vi "MCSA Spectra (1 Motor with IC).vi"(0 "waveforms":waveform(dbl)[](array[waveform]), 2 "reset? (F)":bool, 7 "spectrum settings":T5={"number of lines"=15000, "% overlap"=0.0, "maximum frequency [Hz]"=250.0}, 9 "initial conditions":T1 {"zoom FFT settings"."FFT settings"."window" items=["Rectangle"=0, "Hanning"=1, "Hamming"=2, "Blackman-Harris"=3, "Exact Blackman"=4, "Blackman"=5, "Flat Top"=6, "4 Term B-Harris "=7, "7 Term B-Harris"=8, "Low Sidelobe"=9, "Blackman Nuttall"=11, "Triangle"=30, "Bartlett-Hanning"=31, "Bohman"=32, "Parzen"=33, "Welch"=34, "Kaiser"=60, "Dolph-Chebyshev"=61, "Gaussian"=62]}, 11 "error in (no error)":errorcluster, 12 "demodulation settings":cluster{"enable? (F)":bool, "algorithm":T2}={"enable? (F)"=FALSE, "algorithm"=enum."3-phase signals"}) -> (3 "new spectrum available?":bool, 4 "spectrum information":T4, 10 "final conditions":T1 {"zoom FFT settings"."FFT settings"."window" items=["Rectangle"=0, "Hanning"=1, "Hamming"=2, "Blackman-Harris"=3, "Exact Blackman"=4, "Blackman"=5, "Flat Top"=6, "4 Term B-Harris "=7, "7 Term B-Harris"=8, "Low Sidelobe"=9, "Blackman Nuttall"=11, "Triangle"=30, "Bartlett-Hanning"=31, "Bohman"=32, "Parzen"=33, "Welch"=34, "Kaiser"=60, "Dolph-Chebyshev"=61, "Gaussian"=62]}, 15 "error out":errorcluster)   [LabVIEW 2014, in "NI_EP_Motor Monitoring.lvlib"]
doc: "Calculates the zoom fast Fourier Transform (FFT) spectra of the motor. You must manually select the polymorphic instance you want to use."
uses:
  <vilib>/addons/Electrical Power/Motor Monitoring/NI_EP_Motor Monitoring.lvlib
  <vilib>/addons/Electrical Power/Motor Monitoring/subVIs/ep_Spectra Settings.ctl
  <vilib>/addons/Electrical Power/Motor Monitoring/subVIs/ep_Demodulation Algorithm.ctl
  <vilib>/addons/Electrical Power/Motor Monitoring/subVIs/ep_Initial Conditions for MCSA Spectra.ctl
  <vilib>/addons/Electrical Power/Motor Monitoring/subVIs/ep_Zoom FFT Settings.ctl
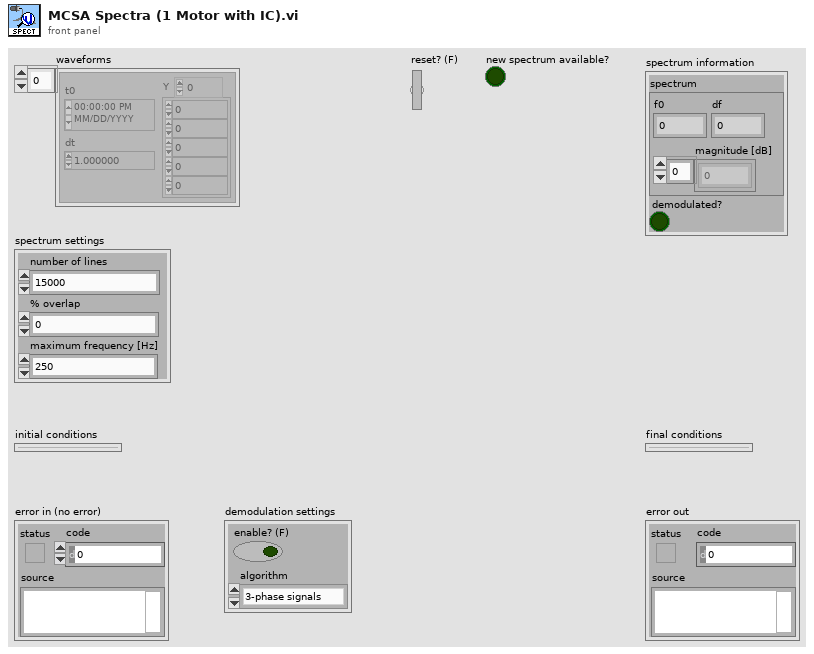
[diagram p1: front panel]
types:
  T1 = typedef "NI_EP_Motor Monitoring.lvlib/ep_Initial Conditions for MCSA Spectra.ctl" = cluster{"hilbert state":cluster{"delay conditions":dbl[], "filter conditions":dbl[]}, "zoom FFT state":cluster{"phase state":dbl, "zoom FFT state":cluster{"zoom settings state":cluster{"zoom":i32, "stop band attenuation":enum16{"84 dB", "96 dB", "120 dB"}, "alias protect in final transition":bool, "oversampling ratio":dbl}, "SML Decimation Filter (complex input) state":cluster{"decimation settings state":cluster{"M":i32, "stop band attenuation":enum16{"84 dB", "96 dB", "120 dB"}, "alias protect in transition band":bool, "oversampling ratio":dbl}, "counter for garbage samples state":i32, "sml_Parameter Setting for Zoom Factor state":cluster{"filter length * interpolation state":i32, "interpolation state":i32, "comb filter order state":i32, "CFIR par state":cluster{"h":dbl[], "M":i32, "N":i32}, "LFIR par state":cluster{"h":dbl[], "M":i32, "N":i32}, "CIC Stages state":i32}, "aal_CIC (complex input) state":cluster{"aal_cascaded moving average (complex input) state":cluster{"states":cdb[], "circular buffers state":cdb[][], "circular buffer counter state":i32}, "aal_moving average with decimation by order (complex input) state":cluster{"residue result state":cdb, "processed data counter state":i32}}, "sml_Cascaded Decimation Filter (complex input) CFIR state":cluster{"unprocessed data state":cdb[], "final conditions state":cdb[][], "sml_M-1 Decimator with IC (complex input) state":cluster{"coefficients in reverse order state":dbl[], "max index for coefficients state":i32}}, "sml_Cascaded Decimation Filter (complex input) LFIR state":cluster{"unprocessed data state":cdb[], "final conditions state":cdb[][], "sml_M-1 Decimator with IC (complex input) state":cluster{"coefficients in reverse order state":dbl[], "max index for coefficients state":i32}}}, "ma_SML Data Packing (complex input) state":cluster{"array getting packed state":cdb[], "last array processed state":cdb[], "index state":i32, "packing parameters state":cluster{i32, "size":i32}}}, "FFT{X} [Vrms]":cdb[]}, "IIR filter state":cluster{"filter state":dbl[]}, "demodulation settings":cluster{"enable? (F)":bool, "algorithm":T2}, "highpass IIR Filter":cluster{"filter structure":enum32{"IIR 2nd Order", "IIR 4th Order"}, "Reverse Coefficients":dbl[], "Forward Coefficients":dbl[]}, "Hilbert FIR filter":cluster{"coefficients":dbl[], "delay":i32}, "zoom FFT settings":T3}
  T2 = typedef "NI_EP_Motor Monitoring.lvlib/ep_Demodulation Algorithm.ctl" = enum16{"1-phase signal", "3-phase signals"}
  T3 = typedef "NI_EP_Motor Monitoring.lvlib/ep_Zoom FFT Settings.ctl" = cluster{"FFT settings":cluster{"window":u16, "Window Size":i32, "FFT Size":i32, "%overlap":dbl}, "zoom settings":cluster{"zoom":i32, "stop band attenuation":enum16{"84 dB", "96 dB", "120 dB"}, "alias protect in final transition":bool, "oversampling ratio":dbl}, "other settings":cluster{"fmod":dbl, "f0":dbl, "df":dbl, "oidx":i32, "olen":i32}, "iterations":i32, "max block size":i32, "fs":dbl}
  T4 = cluster{"spectrum":cluster{"f0":dbl, "df":dbl, "magnitude [dB]":dbl[]}, "demodulated?":bool}
  T5 = typedef "NI_EP_Motor Monitoring.lvlib/ep_Spectra Settings.ctl" = cluster{"number of lines":i32, "% overlap":dbl, "maximum frequency [Hz]":dbl}
  T6 = cluster{"spectra":cluster{"f0":dbl, "df":dbl, "magnitude [dB]":dbl[]}, "demodulated?":bool}
  T7 = cluster{"demodulation settings":cluster{"enable? (F)":bool, "algorithm":T2}, "dt":dbl, "block size":i32}
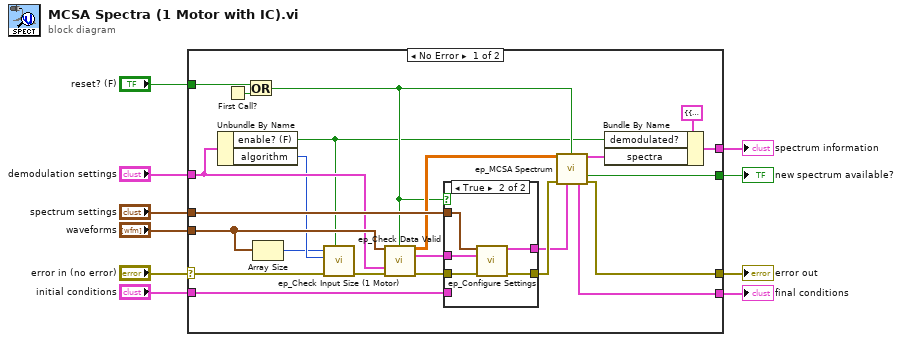
[diagram p0: block diagram]
diagram:
  n1 = case shown="No Error" "error in (no error)" {
    selector: "error in (no error)" -> [w16 w42]
    tunnel: [w30 w42] -> w7
    tunnel: "waveforms" -> [w19 _]
    tunnel: "reset? (F)" -> [w33 _]
    tunnel: "spectrum settings" -> [w27 _]
    tunnel: "demodulation settings" -> [w17 _]
    tunnel: [w31 _] -> w4
    tunnel: [w29 _] -> w3
    tunnel: [w22 w41] -> w2
    tunnel: "initial conditions" -> [w21 w41]
    frame No Error {
      n2 = Unbundle By Name(w17) -> ("enable? (F)"=w11:bool, "algorithm"=w13:T2)
      n3 = First Call?() -> (First Call?: T/F=w32:bool)
      n4 = Or(x=w33, y=w32) -> (x .or. y?=w14:bool)
      n5 = Array Size(array=w19) -> (size(s)=w12:i32)
      n6 = call <vilib>:"ep_Check Input Size (1 Motor).vi"("check? (F)"=w11, "error in (no error)"=w16, "algorithm"=w13, "number of channels"=w12) -> ("error out"=w15:errorcluster)  [unwired: 7 in]
      n7 = call <vilib>:"ep_Check Data Valid.vi"("waveforms"=w19, "reset? (F)"=w14, "demodulation settings"=w17, "error in (no error)"=w15) -> ("signals"=w24:dbl[][], "parameters"=w20:T7, "error out"=w18:errorcluster)  [unwired: 8 in, 1 out]
      n8 = case shown="True" w14 {
        tunnel: [w34 w36] -> w23
        tunnel: w18 -> [w35 w40]
        tunnel: w27 -> [_ w39]
        tunnel: w20 -> [_ w38]
        tunnel: [w35 w37] -> w25
        tunnel: w21 -> [w34 _]
        frame False {
        }
        frame True {
          n9 = call <vilib>:"ep_Configure Settings.vi"("spectra settings"=w39, "parameters"=w38, "error in (no error)"=w40) -> ("initial conditions"=w36:T1, "error out"=w37:errorcluster)  [unwired: 11 in]
        }
      }
      n10 = call <vilib>:"ep_MCSA Spectrum.vi"("signals"=w24, "reset? (F)"=w14, "error in (no error)"=w25, "initial conditions"=w23) -> ("FFT magnitude"=w28:cluster{"f0":dbl, "df":dbl, "spectrum":dbl[]}, "spectrum ready?"=w31:bool, "final conditions"=w22:T1, "error out"=w30:errorcluster)  [unwired: 7 in, 1 out]
      n11 = Bundle By Name(cluster=T6 {"spectra"={"f0"=0.0, "df"=0.0, "magnitude [dB]"=[]}, "demodulated?"=FALSE} ("spectra information"), "demodulated?"=w11, "spectra"=w28) -> (w29:T6)
    }
    frame Error {
    }
  }
  "spectrum information" <- w3
  "new spectrum available?" <- w4
  "error out" <- w7
  "final conditions" <- w2
